vi "Snooze Check Map (SubVI).vi"(7 "Snooze Time (s)":dbl=60.0, 11 "key":string) -> (3 "Snooze Expired?":bool)   [LabVIEW 2019]
doc: "Creates a programmatic method to pause (or snooze) a function for a selected number of seconds (default 60). \n\nThis utility creates a Map that contains a key/value pair. When the function is called, it creates a new map entry based on the provided key name (first call) and stores the current time as the value. Subsequent calls, the utility will check if the snooze time expired and returns TRUE, otherwise it returns FALSE. This is reentrant and can keep track of multiple snooze timers simultaneously. \n\nTypical use case: to limit (email) alert intervals or log entires when thresholds are violated. \n\nNREL 2021"
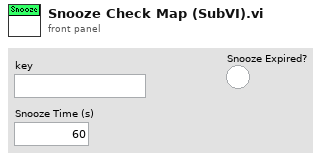
[diagram p1: front panel]
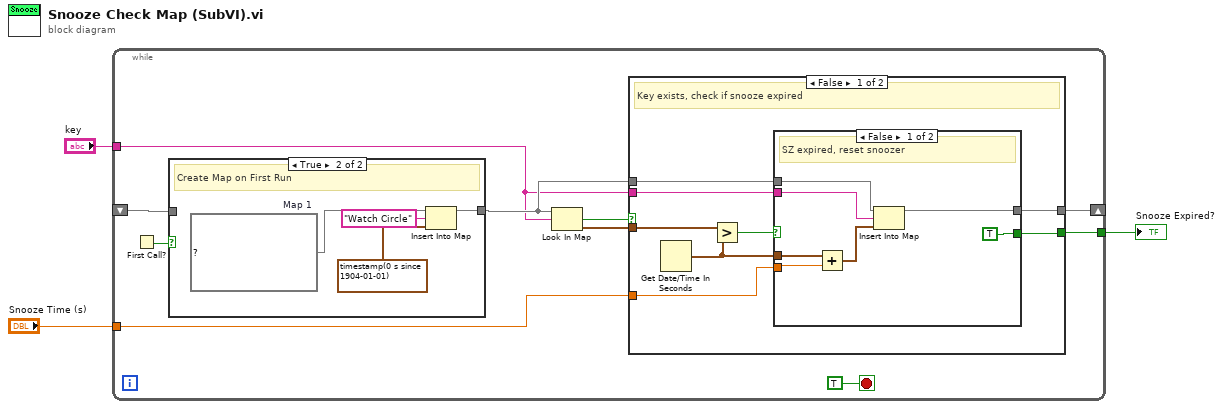
[diagram p0: block diagram]
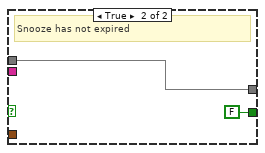
[diagram p2: hidden frame]
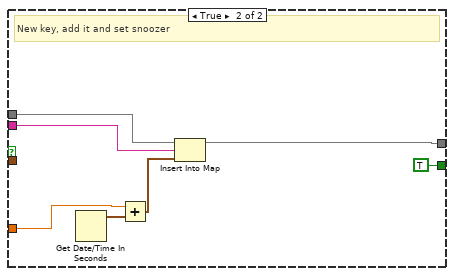
[diagram p3: hidden frame]
diagram:
  n1 = while {
    shift-right: [w5] -> _
    shift-left: _ -> [w12]
    tunnel: "key" -> [w6]
    tunnel: [w8] -> w2
    tunnel: "Snooze Time (s)" -> [w4]
    stop <- TRUE stop-if-true
    n2 = First Call?() -> (First Call?: T/F=w13:bool)
    n3 = case shown="True" w13 {
      tunnel: [w38 w40] -> w7
      tunnel: w12 -> [w38 _]
      frame False {
      }
      frame True {
        w42 = map{string, timestamp} {}  # Map 1
        # "Create Map on First Run"
        n4 = Insert Into Map(map in=w42, key="Watch Circle", value=timestamp(0 s since 1904-01-01)) -> (map out=w40:map{string, timestamp})  [unwired: 2 out]
      }
    }
    n5 = Look In Map(map=w7, key=w6) -> (key not found?=w10:bool, value=w9:timestamp)  [unwired: 1 in]
    n6 = case shown="False" w10 {
      tunnel: w9 -> [w21 _]
      tunnel: [w15 TRUE] -> w8
      tunnel: w7 -> [w19 w37]
      tunnel: w6 -> [w18 w35]
      tunnel: [w16 w36] -> w5
      tunnel: w4 -> [w14 w31]
      frame False {
        # "Key exists, check if snooze expired"
        n7 = Get Date/Time In Seconds() -> (seconds since 1Jan1904=w17:timestamp)
        n8 = Greater?(x=w21, y=w17) -> (0:w20:bool)
        n9 = case shown="False" w20 {
          tunnel: w19 -> [w28 w30]
          tunnel: w18 -> [w27 _]
          tunnel: w17 -> [w23 _]
          tunnel: [w25 w30] -> w16
          tunnel: [TRUE FALSE] -> w15
          tunnel: w14 -> [w22 _]
          frame False {
            # "SZ expired, reset snoozer"
            n10 = Add(x=w23, y=w22) -> (x+y=w26:timestamp)
            n11 = Insert Into Map(map in=w28, key=w27, value=w26) -> (map out=w25:map{string, timestamp})  [unwired: 2 out]
          }
          frame True {
            # "Snooze has not expired"
          }
        }
      }
      frame True {
        # "New key, add it and set snoozer"
        n12 = Get Date/Time In Seconds() -> (seconds since 1Jan1904=w34:timestamp)
        n13 = Add(x=w31, y=w34) -> (x+y=w33:timestamp)
        n14 = Insert Into Map(map in=w37, key=w35, value=w33) -> (map out=w36:map{string, timestamp})  [unwired: 2 out]
      }
    }
  }
  "Snooze Expired?" <- w2
